vi "Init.vi"(6 "InitFlags":T1 items=["NONE"=0, "SDL_INIT_AUDIO"=16, "SDL_INIT_VIDEO"=32, "SDL_INIT_JOYSTICK"=512, "SDL_INIT_HAPTIC"=4096, "SDL_INIT_GAMEPAD"=8192, "SDL_INIT_EVENTS"=16384, "SDL_INIT_SENSOR"=32768, "SDL_INIT_CAMER"=65536], 8 "No Error":errorcluster) -> (0 "error out":errorcluster)   [LabVIEW 2024, in "SDL3.lvlib" / "Init.lvlib"]
doc: "<B>Summary</B>\nInitialize the SDL library.\n\n<B>Remarks</B>\nSDL_Init() simply forwards to calling SDL_InitSubSystem(). Therefore, the two may be used interchangeably. Though for readability of your code SDL_InitSubSystem() might be preferred.\n\nThe file I/O (for example: SDL_IOFromFile) and threading (SDL_CreateThread) subsystems are initialized by default. Message boxes (SDL_ShowSimpleMessageBox) also attempt to work without initializing the video subsystem, in hopes of being useful in showing an error dialog when SDL_Init fails. You must specifically initialize other subsystems if you use them in your application.\n\nLogging (such as SDL_Log) works without initialization, too.\n\nflags may be any of the following OR'd together:\n\nSDL_INIT_AUDIO: audio subsystem; automatically initializes the events subsystem\nSDL_INIT_VIDEO: video subsystem; automatically initializes the events subsystem\nSDL_INIT_JOYSTICK: joystick subsystem; automatically initializes the events subsystem\nSDL_INIT_HAPTIC: haptic (force feedback) subsystem\nSDL_INIT_GAMEPAD: gamepad subsystem; automatically initializes the joystick subsystem\nSDL_INIT_EVENTS: events subsystem\nSDL_INIT_SENSOR: sensor subsystem; automatically initializes the events subsystem\nSDL_INIT_CAMERA: camera subsystem; automatically initializes the events subsystem\nSubsystem initialization is ref-counted, you must call SDL_QuitSubSystem() for each SDL_InitSubSystem() to correctly shutdown a subsystem manually (or call SDL_Quit() to force shutdown). If a subsystem is already loaded then this call will increase the ref-count and return.\n\nConsider reporting some basic metadata about your application before calling SDL_Init, using either SDL_SetAppMetadata() or SDL_SetAppMetadataProperty()."
uses:
  Init.lvlib
  InitFlags--ring.ctl
  Error/Error.lvlib
  Lib/SDL3-32.dll
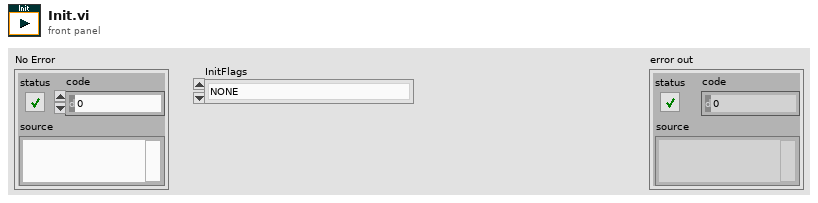
[diagram p1: front panel]
types:
  T1 = typedef "SDL3.lvlib/Init.lvlib/InitFlags--ring.ctl" = u32
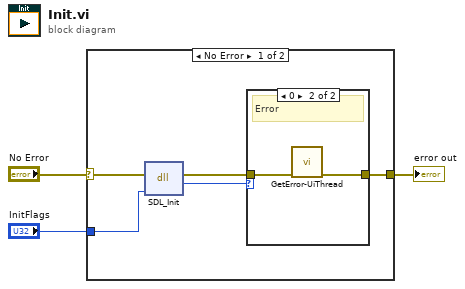
[diagram p0: block diagram]
diagram:
  n1 = case shown="No Error" "No Error" {
    selector: "No Error" -> [w7 w12]
    tunnel: "InitFlags" -> [w8 _]
    tunnel: [w4 w12] -> w2
    frame No Error {
      n2 = dll-call lib="C:/Users/Thomas/Documents/Projects/LV-SDL3/Lib/SDL3-*.*" fn="SDL_Init"(error in=w7, "flags"=w8) -> (error out=w5:errorcluster, "return type"=w6:i32)  [unwired: 3 in, 1 out]
      n3 = case shown="0" w6 {
        tunnel: w5 -> [w9 w11]
        tunnel: [w9 w10] -> w4
        frame Default {
          # "Ok"
        }
        frame 0 {
          # "Error"
          n4 = call "GetError-UiThread.vi"("No Error"=w11) -> ("error out"=w10:errorcluster)  [unwired: 10 in]
        }
      }
    }
    frame Error {
    }
  }
  "error out" <- w2
